vi "Get Subscription Attributes.vi"(8 "error in (no error)":errorcluster, 11 "Subscription in":refnum<class "Subscription.lvclass">) -> (0 "error out":errorcluster, 2 "Subscription Attributes":T1[](array[typedef]), 3 "Subscription out":refnum<class "Subscription.lvclass">)   [LabVIEW 2015, in "NI_AWS_SNS.lvlib" / "Subscription.lvclass"]
uses:
  Subscription.lvclass
  Subscription Attribute Value Pair.ctl
  Subscription Attribute.ctl
  Core/HTTP Request/Request Options.ctl
  Core/HTTP Request/Name Value Pair.ctl
  Core/ARN/ARN.lvclass/ARN.ctl
  Core/ARN/Read ARN.vi
  Core/HTTP Request/HTTP Request.lvclass
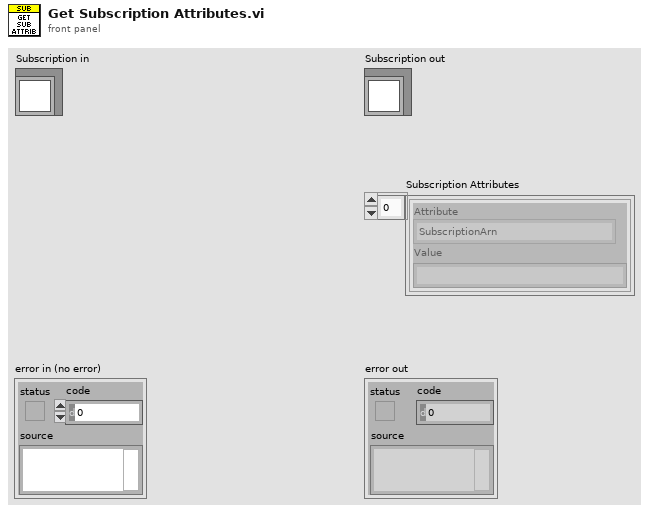
[diagram p1: front panel]
types:
  T1 = typedef "NI_AWS_SNS.lvlib/Subscription.lvclass/Subscription Attribute Value Pair.ctl" = cluster{"Attribute":T2, "Value":string}
  T2 = typedef "NI_AWS_SNS.lvlib/Subscription.lvclass/Subscription Attribute.ctl" = enum16{"SubscriptionArn", "TopicArn", "Owner", "ConfirmationWasAuthenticated", "DeliveryPolicy", "EffectiveDeliveryPolicy", "RawMessageDelivery", "Endpoint", "Protocol"}
  T3 = typedef "NI_AWS_Core.lvlib/HTTP Request.lvclass/Name Value Pair.ctl" = cluster{"name":string, "value":string}
  T4 = typedef "NI_AWS_Core.lvlib/HTTP Request.lvclass/Request Options.ctl" = cluster{"request headers":T3[], "request parameters":T3[], "request body":string}
  T5 = typedef "NI_AWS_Core.lvlib/HTTP Request.lvclass/Response.ctl" = cluster{"Headers":string, "Body":string}
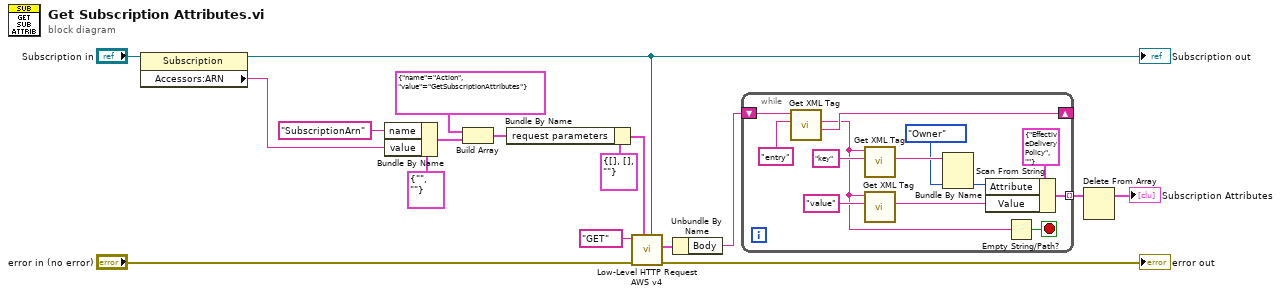
[diagram p0: block diagram]
diagram:
  n1 = property class="Subscription"(reference="Subscription in") -> (reference out=w2:refnum<class "Subscription.lvclass">, "Accessors:ARN"=w1:string)  [unwired: 1 in, 1 out]
  "Subscription out" <- w2
  n2 = Bundle By Name(cluster=T3 {"name"="", "value"=""} ("Name Value Pair"), "name"="SubscriptionArn", "value"=w1) -> (w4:T3)
  n3 = Build Array(T3 {"name"="Action", "value"="GetSubscriptionAttributes"} ("Name Value Pair"), w4) -> (w7:T3[])
  n4 = Bundle By Name(cluster=T4 {"request headers"=[], "request parameters"=[], "request body"=""} ("Request Options"), "request parameters"=w7) -> (w15:T4)
  n5 = call "Low-Level HTTP Request AWS v4.vi"("AWS Core"=w2, "Request Options"=w15, "error in (no error)"="error in (no error)", "HTTP-Verb"="GET") -> ("error out"=→"error out":errorcluster, "Response"=w14:T5)  [unwired: 5 in, 1 out]
  n6 = Unbundle By Name(w14) -> ("Body"=w13:string)
  n7 = while {
    shift-right: [w29] -> _
    shift-left: w13 -> [w30]
    tunnel: [w24] -> w12 mode=indexing
    stop <- w22 stop-if-true
    n8 = call "Get XML Tag.vi"("Tag name"="entry", "XML String in"=w30) -> ("Remaining string"=w29:string, "Tag value"=w23:string)  [unwired: 5 in, 3 out]
    n9 = call "Get XML Tag.vi"("Tag name"="key", "XML String in"=w23) -> ("Tag value"=w21:string)  [unwired: 5 in, 4 out]
    n10 = call "Get XML Tag.vi"("Tag name"="value", "XML String in"=w23) -> ("Tag value"=w25:string)  [unwired: 5 in, 4 out]
    n11 = Scan From String(input string=w21, default 1=Subscription_Attribute."Owner" ("Attribute")) -> (output 1=w20:T2)  [unwired: 3 in, 3 out]
    n12 = Bundle By Name(cluster=T1 {"Attribute"=enum."EffectiveDeliveryPolicy", "Value"=""} ("Subscription Attribute Value Pair"), "Attribute"=w20, "Value"=w25) -> (w24:T1)
    n13 = Empty String/Path?(string/path=w23) -> (empty?=w22:bool)
  }
  n14 = Delete From Array(array=w12) -> (array with subset deleted=→"Subscription Attributes":T1[])  [unwired: 2 in, 1 out]
